vi "WriteSyncInfoRequest.vi"(8 "error in (no error)":errorcluster, 10 "SyncInfo":variant, 11 "ModuleID":i32) -> (0 "error out":errorcluster)   [LabVIEW 2014, in "DigitizerPlugins.lvlib" / "DigitizerBase.lvclass"]
uses:
  DigitizerBase.lvclass
  DigitizerModule/Protected/clEventType.ctl
  <vilib>/Utility/error.llb/Error Cluster From Error Code.vi
  <vilib>/ErrorRing/Error Ring.xnode
  DigitizerModule/DigitizerModule.lvlib
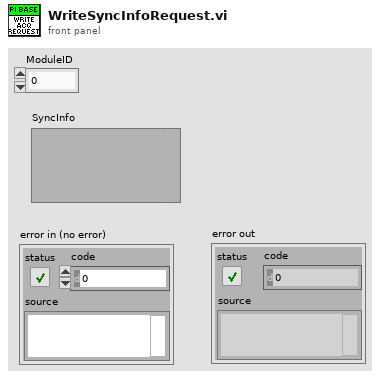
[diagram p1: front panel]
types:
  T1 = typedef "DigitizerModule.lvlib/clRequestEvents.ctl" = cluster{"StopRequest":refnum<user-event>, "PathToINI":refnum<user-event>, " LoadPlugin":refnum<user-event>, "ShowPanel":refnum<user-event>, "PrefDlg":refnum<user-event>, "ReadChannels":refnum<user-event>, "WriteChannels":refnum<user-event>, "ConfigChannels":refnum<user-event>, "ReadAcq":refnum<user-event>, "WriteAcq":refnum<user-event>, "ConfigAcq":refnum<user-event>, "ReadTriggers":refnum<user-event>, "WriteTriggers":refnum<user-event>, "ConfigTriggers":refnum<user-event>, "FetchWfrm":refnum<user-event>, "ReadWfrm":refnum<user-event>, "Initialize":refnum<user-event>, "Abort":refnum<user-event>, "ReadSyncInfo":refnum<user-event>, "WriteSyncInfo":refnum<user-event>}
  T2 = typedef "DigitizerModule.lvlib/clEventType.ctl" = cluster{"ModuleID":i32, "Data":variant}
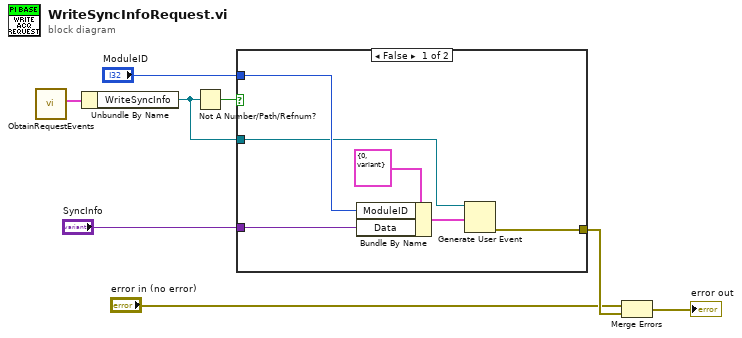
[diagram p0: block diagram]
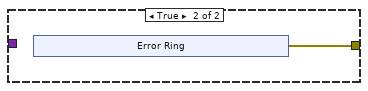
[diagram p2: hidden frame]
diagram:
  n1 = call "ObtainRequestEvents.vi"() -> ("clDigitizerRequestEvents"=w8:T1)  [unwired: 10 in, 1 out]
  n2 = Unbundle By Name(w8) -> ("WriteSyncInfo"=w6:refnum<user-event>)
  n3 = Not A Number/Path/Refnum?(number/path/refnum=w6) -> (NaN/Path/Refnum?=w7:bool)
  n4 = case shown="False" w7 {
    tunnel: w6 -> [w11 _]
    tunnel: "ModuleID" -> [w13 _]
    tunnel: [w10 w15] -> w3
    tunnel: "SyncInfo" -> [w9 _]
    frame False {
      n5 = Bundle By Name(cluster=T2 {"ModuleID"=0, "Data"=variant} ("clEventType"), "ModuleID"=w13, "Data"=w9) -> (w12:T2)
      n6 = Generate User Event(user event=w11, event data cluster=w12) -> (error out=w10:errorcluster)  [unwired: 2 in, 1 out]
    }
    frame True {
      n7 = xnode "Error Ring"() -> ("error out"=w15:errorcluster)
    }
  }
  n8 = Merge Errors("error in (no error)", w3) -> (→"error out":errorcluster)
